vi "UIWriteCtrl.vi"(4 "UI Flag":string="UI_", 5 "Value Signaling (F)":bool, 6 "Search Whole Word (T)":bool=TRUE, 7 "Class_Hierarchy (F)":bool, 8 "error in":errorcluster, 9 "Control Value":variant, 10 "Control Label":string, 11 "UI Ref cluster in":T1) -> (0 "error out":errorcluster, 3 "UI Ref cluster out":T1)   [LabVIEW 2025, in "UI_Library.lvlib" / "UI_Library.lvclass"]
doc: "Write new value to a Control if found"
uses:
  UI_Library.lvclass
  Controls/UI_RefCluster.ctl
  <vilib>/Utility/Data Type/Type Definitions/Data Type.ctl
  <vilib>/Utility/Data Type/NI_Data Type.lvlib
  UI_Library.lvlib
panel:
  in  "CheckValueChange? (F)":bool
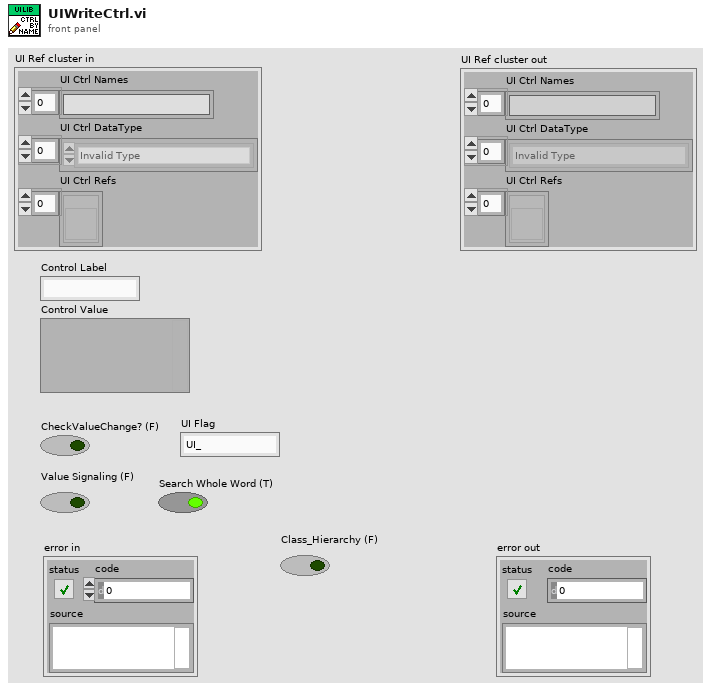
[diagram p1: front panel]
types:
  T1 = typedef "UI_Library.lvlib/UI_RefCluster.ctl" = cluster{"UI Ctrl Names":string[], "UI Ctrl DataType":T2[], "UI Ctrl Refs":refnum<vi>[]}
  T2 = typedef "NI_Data Type.lvlib/Data Type.ctl" = enum8{"Invalid Type", "Void", "I8", "I16", "I32", "I64", "U8", "U16", "U32", "U64", "Single Float", "Double Float", "Extended Float", "Single Complex", "Double Complex", "Extended Complex", "Enum U8", "Enum U16", "Enum U32", "Enum U64", "Single Float With Unit", "Double Float With Unit", "Extended Float With Unit", "Single Complex with Unit", "Double Complex with Unit", "Extended Complex with Unit", "Boolean", "String", "Path", "Picture", "Tag", "Array", "Cluster", "Variant", "LV Variant", "Waveform", "Timestamp", "Digital Waveform", "Digital Data", "ExpressData", "Refnum", "External Data", "VI", "Poly VI", "LabVIEW Class Instance", "Fixed Point", "Set Collection", "Map Collection"}
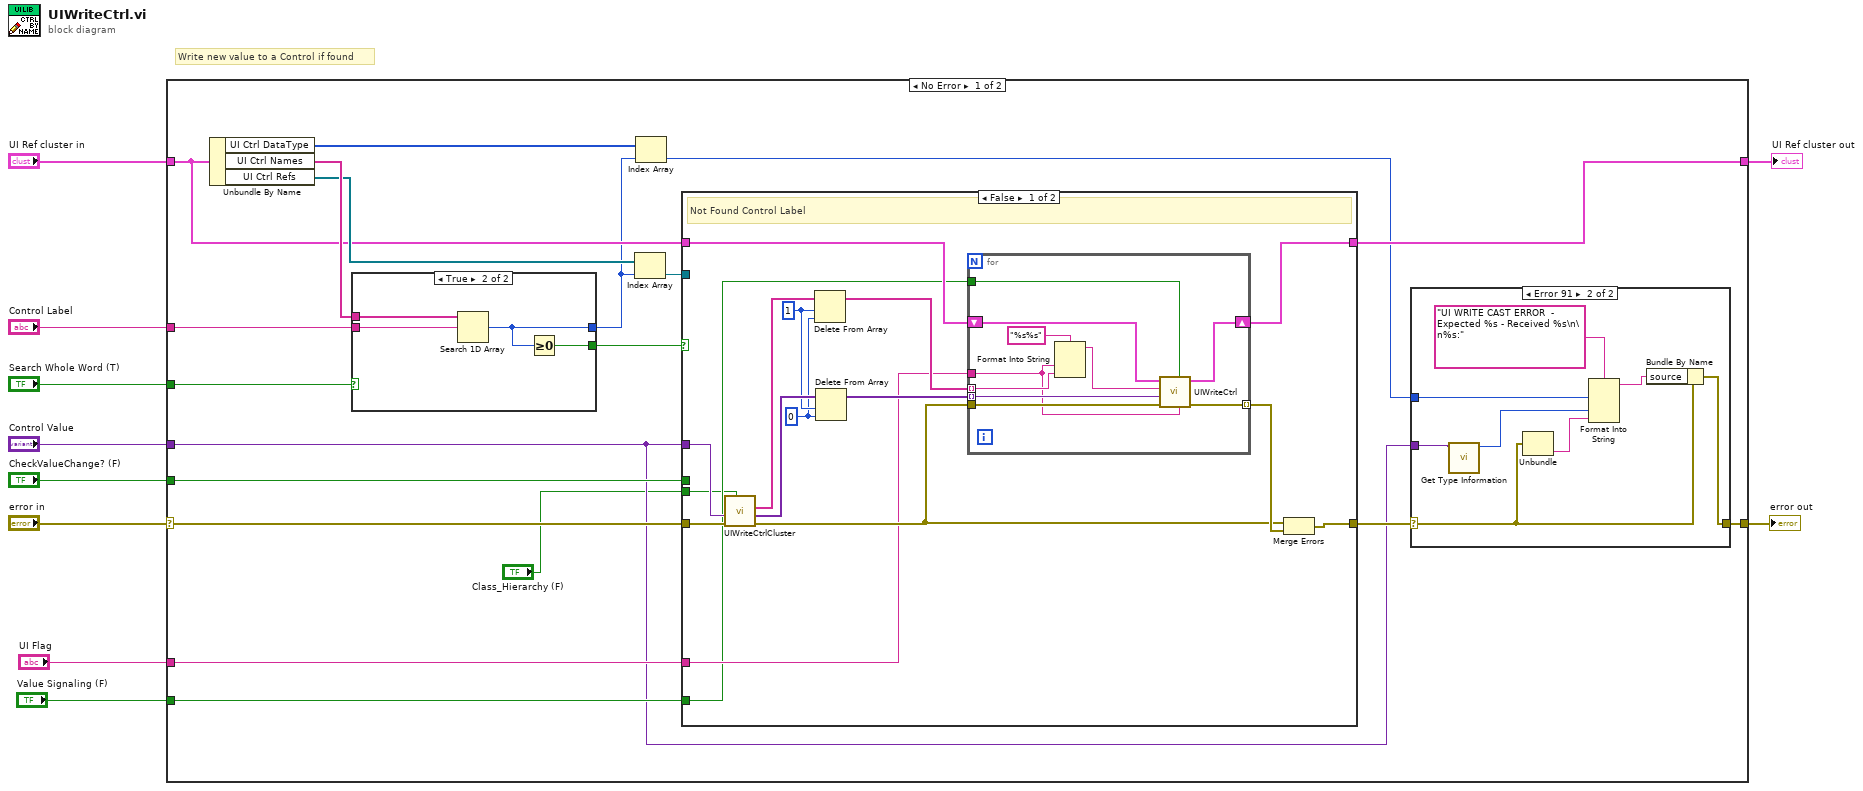
[diagram p0: block diagram]
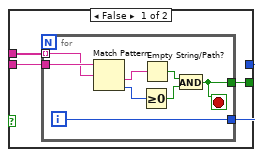
[diagram p2: hidden frame]
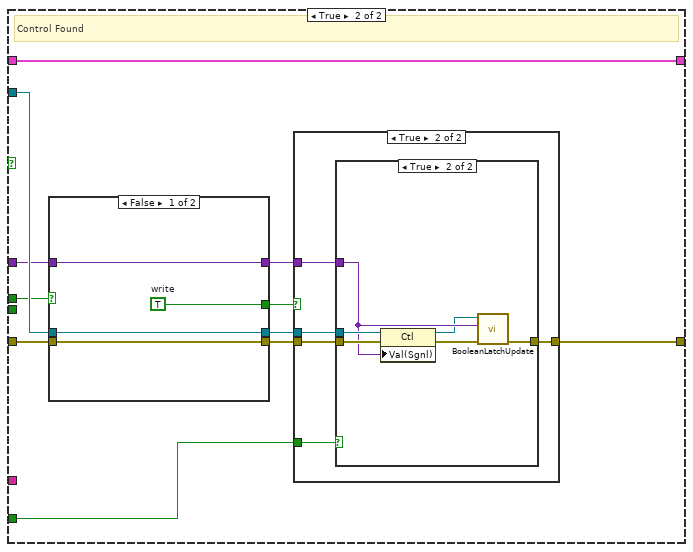
[diagram p3: hidden frame]
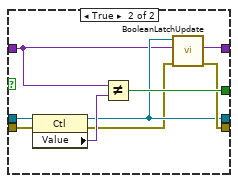
[diagram p4: hidden frame]
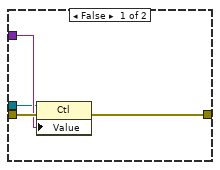
[diagram p6: hidden frame]
diagram:
  # "Write new value to a Control if found"
  n1 = case shown="No Error" "error in" {
    selector: "error in" -> [w26 w122]
    tunnel: [w18 w122] -> w10
    tunnel: "Control Value" -> [w12 _]
    tunnel: "Control Label" -> [w22 _]
    tunnel: [w21 w121] -> w6
    tunnel: "UI Ref cluster in" -> [w20 w121]
    tunnel: "CheckValueChange? (F)" -> [w25 _]
    tunnel: "Search Whole Word (T)" -> [w23 _]
    tunnel: "Value Signaling (F)" -> [w14 _]
    tunnel: "UI Flag" -> [w13 _]
    frame No Error {
      n2 = Unbundle By Name(w20) -> ("UI Ctrl DataType"=w16:T2[], "UI Ctrl Names"=w29:string[], "UI Ctrl Refs"=w28:refnum<vi>[])
      n3 = case shown="True" w23 {
        tunnel: w29 -> [w32 w45]
        tunnel: w22 -> [w33 w44]
        tunnel: [w31 w43] -> w17
        tunnel: [w30 w42] -> w24
        frame False {
          n4 = for {
            tunnel: w33 -> [w41]
            tunnel: w32 -> [w40] mode=indexing
            tunnel: [w38] -> w31
            tunnel: [w34] -> w30
            i -> [w38]
            stop <- w34 stop-if-true
            n5 = Match Pattern(string=w41, regular expression=w40) -> (after substring=w37:string, offset past match=w39:i32)  [unwired: 1 in, 2 out]
            n6 = Greater Or Equal To 0?(x=w39) -> (x >= 0?=w35:bool)
            n7 = Empty String/Path?(string/path=w37) -> (empty?=w36:bool)
            n8 = And(x=w36, y=w35) -> (x .and. y?=w34:bool)
          }
        }
        frame True {
          n9 = Search 1D Array(1D array=w45, element=w44) -> (index of element=w43:i32)  [unwired: 1 in]
          n10 = Greater Or Equal To 0?(x=w43) -> (x >= 0?=w42:bool)
        }
      }
      n11 = Index Array(array=w28, index=w17) -> (element=w27:refnum<vi>)
      n12 = Index Array(array=w16, index=w17) -> (element=w15:T2)
      n13 = case shown="False" w24 {
        tunnel: w27 -> [_ w81]
        tunnel: w26 -> [w61 w80]
        tunnel: [w51 w82] -> w19
        tunnel: w12 -> [w56 w73]
        tunnel: w25 -> [_ w76]
        tunnel: [w52 w74] -> w21
        tunnel: w20 -> [w55 w74]
        tunnel: w13 -> [w48 _]
        tunnel: w14 -> [w47 w72]
        tunnel: "Class_Hierarchy (F)" -> [w46 _]
        frame False {
          w57 = 0 ("index")
          w58 = 1 ("length")
          # "Not Found Control Label"
          n14 = call "UIWriteCtrlCluster.vi"("Class_Hierarchy (F)"=w46, "error in"=w61, "Control Value"=w56) -> ("error out"=w50:errorcluster, "NestedCtrlValues"=w59:variant[], "NestedCtrlNames"=w60:string[])  [unwired: 6 in]
          n15 = Delete From Array(array=w60, length=w58, index=w57) -> (array with subset deleted=w49:string[])  [unwired: 1 out]
          n16 = Delete From Array(array=w59, length=w58, index=w57) -> (array with subset deleted=w54:variant[])  [unwired: 1 out]
          n17 = for {
            tunnel: w49 -> [w64] mode=indexing
            tunnel: w54 -> [w67] mode=indexing
            shift-right: [w70] -> w52
            shift-left: w55 -> [w71]
            tunnel: w50 -> [w69]
            tunnel: [w68] -> w53 mode=indexing
            tunnel: w48 -> [w63]
            tunnel: w47 -> [w62]
            n18 = Format Into String(format string="%s%s", w63, w64) -> (resulting string=w65:string)  [unwired: 2 in, 1 out]
            n19 = call "UIWriteCtrl.vi"("UI Flag"=w63, "Value Signaling (F)"=w62, "error in"=w69, "Control Value"=w67, "Control Label"=w65, "UI Ref cluster in"=w71) -> ("error out"=w68:errorcluster, "UI Ref cluster out"=w70:T1)  [unwired: 4 in]
          }
          n20 = Merge Errors(w50, w53) -> (w51:errorcluster)
        }
        frame True {
          # "Control Found"
          n21 = case shown="False" w76 {
            tunnel: w81 -> [w84 w95]
            tunnel: w80 -> [w85 w91]
            tunnel: w73 -> [w86 w89]
            tunnel: [w84 w90] -> w79
            tunnel: [w85 w92] -> w78
            tunnel: [w83 w94] -> w77
            tunnel: [w86 w88] -> w75
            frame False {
              w83 = TRUE  # write
            }
            frame True {
              n22 = property on="Property Node" class="Ctl"(reference=w95, error in=w91) -> (reference out=w90:refnum<vi>, error out=w87:errorcluster, "Value"=w93:variant)
              n23 = Not Equal?(x=w89, y=w93) -> (x != y?=w94:bool)
              n24 = call "BooleanLatchUpdate.vi"("error in"=w87, "Control Value in"=w89, "Control in"=w90) -> ("error out"=w92:errorcluster, "Control Value out"=w88:variant)  [unwired: 7 in]
            }
          }
          n25 = case shown="True" w77 {
            tunnel: [w96 w101] -> w82
            tunnel: w75 -> [_ w100]
            tunnel: w79 -> [_ w99]
            tunnel: w78 -> [w96 w98]
            tunnel: w72 -> [_ w97]
            frame False {
            }
            frame True {
              n26 = case shown="True" w97 {
                tunnel: [w105 w106] -> w101
                tunnel: w100 -> [w103 w109]
                tunnel: w99 -> [w102 w111]
                tunnel: w98 -> [w104 w110]
                frame False {
                  n27 = property on="Property Node" class="Ctl"(reference=w102, error in=w104, "Value"=w103) -> (error out=w105:errorcluster)  [unwired: 1 out]
                }
                frame True {
                  n28 = property on="Property Node" class="Ctl"(reference=w111, error in=w110, "Val(Sgnl)"=w109) -> (reference out=w108:refnum<vi>, error out=w107:errorcluster)
                  n29 = call "BooleanLatchUpdate.vi"("error in"=w107, "Control Value in"=w109, "Control in"=w108) -> ("error out"=w106:errorcluster)  [unwired: 7 in, 1 out]
                }
              }
            }
          }
        }
      }
      n30 = case shown="Error 91" w19 {
        selector: w19 -> [w112 w117]
        tunnel: [w112 w119] -> w18
        tunnel: w15 -> [_ w116]
        tunnel: w12 -> [_ w113]
        frame #0 {
        }
        frame #1 {
          n31 = call <vilib>:"Get Type Information.vi"("variant"=w113) -> ("type"=w114:T2)  [unwired: 6 in, 4 out]
          n32 = Unbundle(w117) -> ("source"=w115:string)  [unwired: 2 out]
          n33 = Format Into String(format string="UI WRITE CAST ERROR  - Expected %s - Received %s\n\n%s:", w116, w114, w115) -> (resulting string=w118:string)  [unwired: 2 in, 1 out]
          n34 = Bundle By Name(cluster=w117, "source"=w118) -> (w119:errorcluster)
        }
      }
    }
    frame Error {
    }
  }
  "error out" <- w10
  "UI Ref cluster out" <- w6
